vi "TestVI.vi"() -> ()   [LabVIEW 2017]
panel:
  out "String":string
  out "Random":dbl
  in  "stop":bool
  out "current time":timestamp
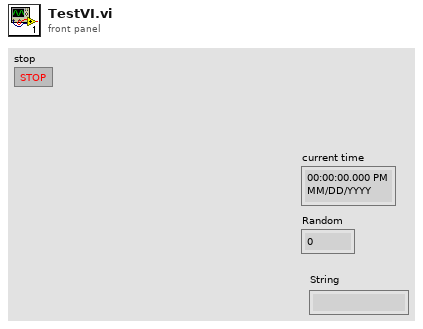
[diagram p1: front panel]
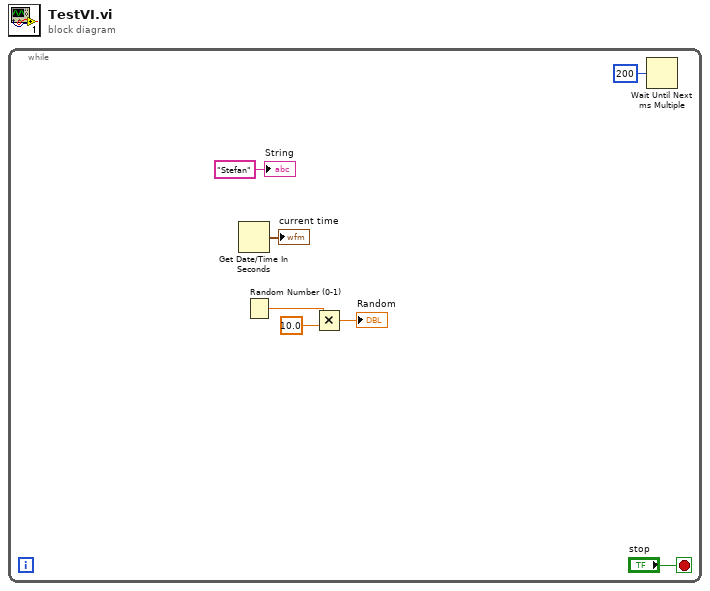
[diagram p0: block diagram]
diagram:
  n1 = while {
    stop <- "stop" stop-if-true
    n2 = Get Date/Time In Seconds() -> (seconds since 1Jan1904=→"current time":timestamp)
    n3 = Random Number (0-1)() -> (number: 0 to 1=w4:dbl)
    n4 = Multiply(x=w4, y=10.0) -> (x*y=→"Random":dbl)
    n5 = Wait Until Next ms Multiple(millisecond multiple=u32 200) -> ()  [unwired: 1 out]
    "String" <- "Stefan" ("String")
  }
